vi "Obtain Broadcast Events.vi"(8 "error in":errorcluster, 10 "Create New? (F)":bool) -> (0 "error out":errorcluster, 2 "DAQ AI Broadcast Events":T1)   [LabVIEW 2020, in "DAQ AI.lvlib"]
doc: "This VI Obtains/Creates the Broadcast events that will be used for other modules to register to receive messages from the module that owns this VI.\n\n<b>NOTE</b>: The contents of this VI are automatically generated and modified by the <b>Tools > DQMH Consortium > DQMH</b> utilities. Consider using those utilities instead of making your own modifications to this VI.\n_____\nBased on DQMH Dev Tools: Project Template 7.1.2.1547."
uses:
  DAQ AI.lvlib
  Broadcast Events--cluster.ctl
  Did Init Argument--cluster.ctl
  Status Updated Argument--cluster.ctl
  Error Reported Argument--cluster.ctl
  Stop Argument--cluster.ctl
  Get Module Execution Status Argument--cluster.ctl
  Send Acquired Data Argument--cluster.ctl
  Clear DAQ Task Argument--cluster.ctl
panel:
  # "NOTE: The contents of this VI are automatically generated and modified by the Tools > DQMH Consortium > DQMH utilities. Consider using those utilities instead of making your own modifications to this VI."
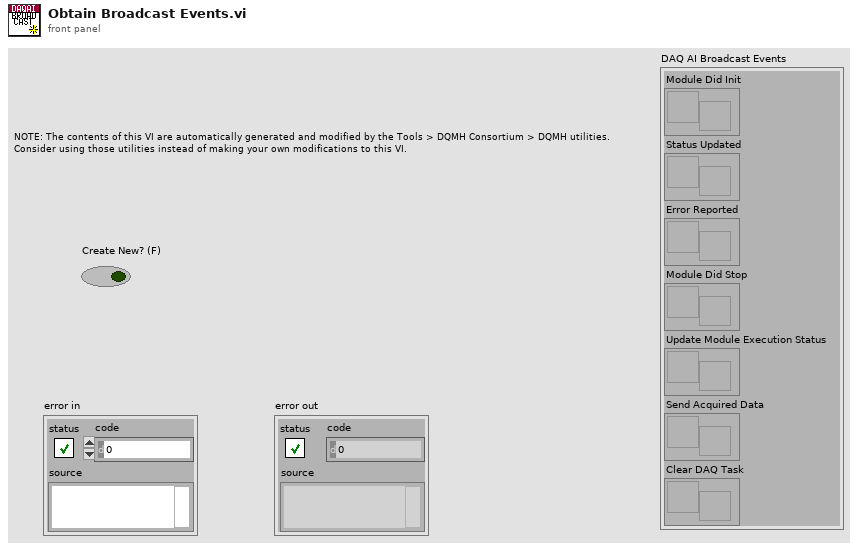
[diagram p1: front panel]
types:
  T1 = typedef "DAQ AI.lvlib/Broadcast Events--cluster.ctl" = cluster{"Module Did Init":refnum<user-event>, "Status Updated":refnum<user-event>, "Error Reported":refnum<user-event>, "Module Did Stop":refnum<user-event>, "Update Module Execution Status":refnum<user-event>, "Send Acquired Data":refnum<user-event>, "Clear DAQ Task":refnum<user-event>}
  T2 = typedef "DAQ AI.lvlib/Clear DAQ Task Argument--cluster.ctl" = cluster{"Module ID":i32, "Dummy":bool}
  T3 = typedef "DAQ AI.lvlib/Send Acquired Data Argument--cluster.ctl" = cluster{"Module ID":i32, "Value":dbl}
  T4 = typedef "DAQ AI.lvlib/Get Module Execution Status Argument--cluster.ctl" = cluster{"Module ID":i32, "Running?":bool}
  T5 = typedef "DAQ AI.lvlib/Stop Argument--cluster.ctl" = cluster{"Module ID":i32, "Origin":string, "Exit via Stop Module Req?":bool, "Wait for Module to stop?":bool}
  T6 = typedef "DAQ AI.lvlib/Error Reported Argument--cluster.ctl" = cluster{"Error":errorcluster, "Additional Information":string, "Module ID":i32, "Module Name":string}
  T7 = typedef "DAQ AI.lvlib/Status Updated Argument--cluster.ctl" = cluster{"Status":string, "Module ID":i32}
  T8 = typedef "DAQ AI.lvlib/Did Init Argument--cluster.ctl" = cluster{"Init?":bool, "Info":string, "Module ID":i32}
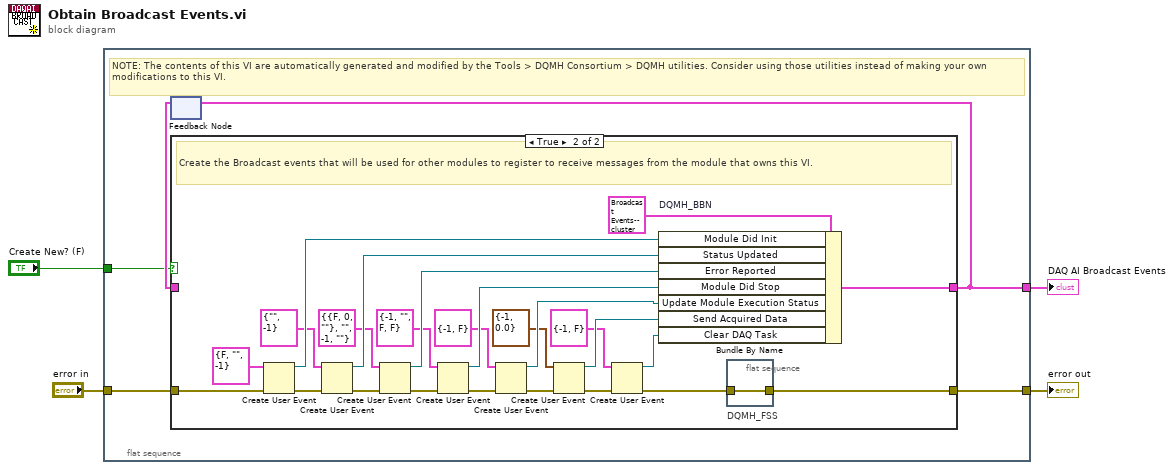
[diagram p0: block diagram]
diagram:
  n1 = flat-sequence {
    tunnel: [w9] -> w4
    tunnel: "error in" -> [w8]
    tunnel: [w6] -> w2
    tunnel: "Create New? (F)" -> [w5]
    frame #0 {
      # "NOTE: The contents of this VI are automatically generated and modified by the Tools > DQMH Consortium > DQMH utilities. Consider using those utilities instead of making your own modifications to this VI."
      n2 = feedback #1() -> (w7:T1)  [unwired: 1 in]
      n3 = case shown="True" w5 {
        tunnel: [w10 w21] -> w9
        tunnel: w8 -> [w10 w36]
        tunnel: [w11 w33] -> w6
        tunnel: w7 -> [w11 _]
        frame False {
          # "Obtain the Broadcast events that were created in a previous call to this VI."
        }
        frame True {
          # "Create the Broadcast events that will be used for other modules to register to receive messages from the module that owns this VI."
          n4 = Create User Event(user event datatype=T8 {"Init?"=FALSE, "Info"="", "Module ID"=-1} ("Did Init Argument"), error in=w36) -> (user event=w34:refnum<user-event>, error out=w31:errorcluster)
          n5 = Create User Event(user event datatype=T7 {"Status"="", "Module ID"=-1} ("Status Updated Argument"), error in=w31) -> (user event=w28:refnum<user-event>, error out=w30:errorcluster)
          n6 = Create User Event(user event datatype=T6 {"Error"={"status"=FALSE, "code"=0, "source"=""}, "Additional Information"="", "Module ID"=-1, "Module Name"=""} ("Error Reported Argument"), error in=w30) -> (user event=w25:refnum<user-event>, error out=w27:errorcluster)
          n7 = Create User Event(user event datatype=T5 {"Module ID"=-1, "Origin"="", "Exit via Stop Module Req?"=FALSE, "Wait for Module to stop?"=FALSE} ("Stop Argument"), error in=w27) -> (user event=w23:refnum<user-event>, error out=w22:errorcluster)
          n8 = Create User Event(user event datatype=T4 {"Module ID"=-1, "Running?"=FALSE} ("Get Module Execution Status Argument"), error in=w22) -> (user event=w19:refnum<user-event>, error out=w20:errorcluster)
          n9 = Create User Event(user event datatype=T3 {"Module ID"=-1, "Value"=0.0} ("Send Acquired Data Argument"), error in=w20) -> (user event=w16:refnum<user-event>, error out=w17:errorcluster)
          n10 = Create User Event(user event datatype=T2 {"Module ID"=-1, "Dummy"=FALSE} ("Clear DAQ Task Argument"), error in=w17) -> (user event=w13:refnum<user-event>, error out=w14:errorcluster)
          n11 = Bundle By Name "DQMH_BBN"(cluster=T1 {"Module Did Init"=refnum, "Status Updated"=refnum, "Error Reported"=refnum, "Module Did Stop"=refnum, "Update Module Execution Status"=refnum, "Send Acquired Data"=refnum, "Clear DAQ Task"=refnum} ("output cluster"), "Module Did Init"=w34, "Status Updated"=w28, "Error Reported"=w25, "Module Did Stop"=w23, "Update Module Execution Status"=w19, "Send Acquired Data"=w16, "Clear DAQ Task"=w13) -> (w33:T1)
          n12 = flat-sequence "DQMH_FSS" {
            tunnel: w14 -> [w37]
            tunnel: [w37] -> w21
            frame #0 {
            }
          }
        }
      }
      n13 = feedback-in #1(w6) -> ()
    }
  }
  "DAQ AI Broadcast Events" <- w2
  "error out" <- w4
